vi "macro_HolDrvController_Execute.vi"   [LabVIEW 2019, in "Trajectory_Library.lvlib"]
uses:
  Trajectory_Library.lvlib
types:
  T1 = typedef "Trajectory_Library.lvlib/PID_TUNING.ctl" = cluster{"Kp":dbl, "Ki":dbl, "Kd":dbl, "MaximumIntegral":dbl, "MinimumIntegral":dbl}
  T2 = typedef "Trajectory_Library.lvlib/PROFILED_PID_CONTROLLER.ctl" = cluster{"Controller":T3, "Goal":T4, "Setpoint":T4, "Constraint":T5}
  T3 = typedef "Trajectory_Library.lvlib/PID_CONTROLLER.ctl" = cluster{"Kp":dbl, "Ki":dbl, "Kd":dbl, "Period":dbl, "Max_Integral":dbl, "Min_Integral":dbl, "Max_Input":dbl, "Min_Input":dbl, "Continuous":bool, "PositionError":dbl, "VelocityError":dbl, "PrevError":dbl, "TotalError":dbl, "PositionTolerance":dbl, "VelocityTolerance":dbl, "SetPoint":dbl, "Kf":dbl, "Prev_Deriv":dbl, "Prev_Deriv 2":dbl, "DerivativeFilter":bool, "Min_Output":dbl, "Max_Output":dbl, "Prev_F_P":dbl, "Prev_F_P_2":dbl, "AntiWindupActive":bool, "Measurement":dbl}
  T4 = typedef "Trajectory_Library.lvlib/TRAPEZOID_PROFILE_STATE.ctl" = cluster{"Position":dbl, "Velocity":dbl}
  T5 = typedef "Trajectory_Library.lvlib/TRAPEZOID_PROFILE_CONSTRAINT.ctl" = cluster{"MaxVelocity":dbl, "MaxAcceleration":dbl}
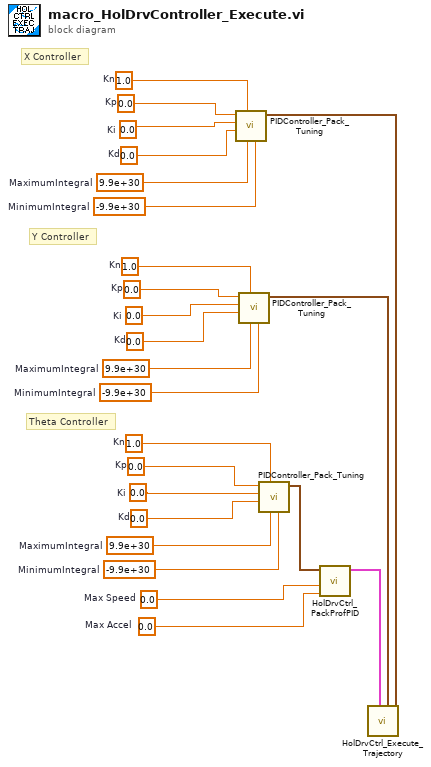
[diagram p0: block diagram]
diagram:
  w16 = 1.0  # Kn
  w13 = 0.0  # Kp
  w4 = 0.0  # Ki
  w3 = 0.0  # Kd
  w2 = 9.9e+30  # MaximumIntegral
  w1 = -9.9e+30  # MinimumIntegral
  w18 = 1.0  # Kn
  w15 = 0.0  # Kp
  w12 = 0.0  # Ki
  w11 = 0.0  # Kd
  w10 = 9.9e+30  # MaximumIntegral
  w9 = -9.9e+30  # MinimumIntegral
  w17 = 1.0  # Kn
  w14 = 0.0  # Kp
  w8 = 0.0  # Ki
  w7 = 0.0  # Kd
  w6 = 9.9e+30  # MaximumIntegral
  w5 = -9.9e+30  # MinimumIntegral
  w19 = 0.0  # Max Accel
  w20 = 0.0  # Max Speed
  # "Theta Controller"
  # "Y Controller"
  # "X Controller"
  n1 = call "PIDController_Pack_Tuning.vi"("MinimumIntegral"=w9, "MaximumIntegral"=w10, "Kn"=w18, "Kd"=w11, "Ki"=w12, "Kp"=w15) -> ("PID Tuning"=w24:T1)  [unwired: 5 in]
  n2 = call "PIDController_Pack_Tuning.vi"("MinimumIntegral"=w5, "MaximumIntegral"=w6, "Kn"=w17, "Kd"=w7, "Ki"=w8, "Kp"=w14) -> ("PID Tuning"=w23:T1)  [unwired: 5 in]
  n3 = call "PIDController_Pack_Tuning.vi"("MinimumIntegral"=w1, "MaximumIntegral"=w2, "Kn"=w16, "Kd"=w3, "Ki"=w4, "Kp"=w13) -> ("PID Tuning"=w21:T1)  [unwired: 5 in]
  n4 = call "HolDrvCtrl_PackProfPID.vi"("Max Accel"=w19, "Max Speed"=w20, "Theta PID Tuning"=w21) -> ("Theta PID CONTROLLER"=w22:T2)  [unwired: 8 in]
  n5 = call "HolDrvCtrl_Execute_Trajectory.vi"("X PID Tuning"=w24, "Y PID Tuning"=w23, "thetaProfiledPID_CTRL"=w22) -> ()  [unwired: 6 in, 3 out]
